vi "Save Image.vi"(8 "error in (no error)":errorcluster, 9 "Export Style":enum32{"Raw", "Graph", "Gray"}(radio), 10 "Export Name":string, 11 "Base Graph in":refnum<class "Base Graph.lvclass">) -> (0 "error out":errorcluster, 3 "Base Graph out":refnum<class "Base Graph.lvclass">)   [LabVIEW 2023, in "Base Graph.lvclass"]
uses:
  Base Graph.lvclass
  Base Graph.lvclass/Base Graph.ctl
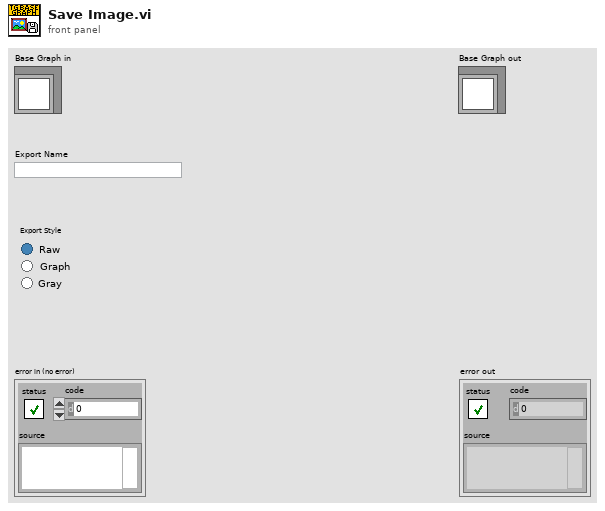
[diagram p1: front panel]
types:
  T1 = typedef "IMAQ Image.ctl" = refnum<image>
  T2 = typedef "imagedata.ctl" = cluster{"image type":i32, "image depth":i32, "image":u8[], "mask":u8[], "colors":u32[], "Rectangle":cluster{"left":i16, "top":i16, "right":i16, "bottom":i16}}
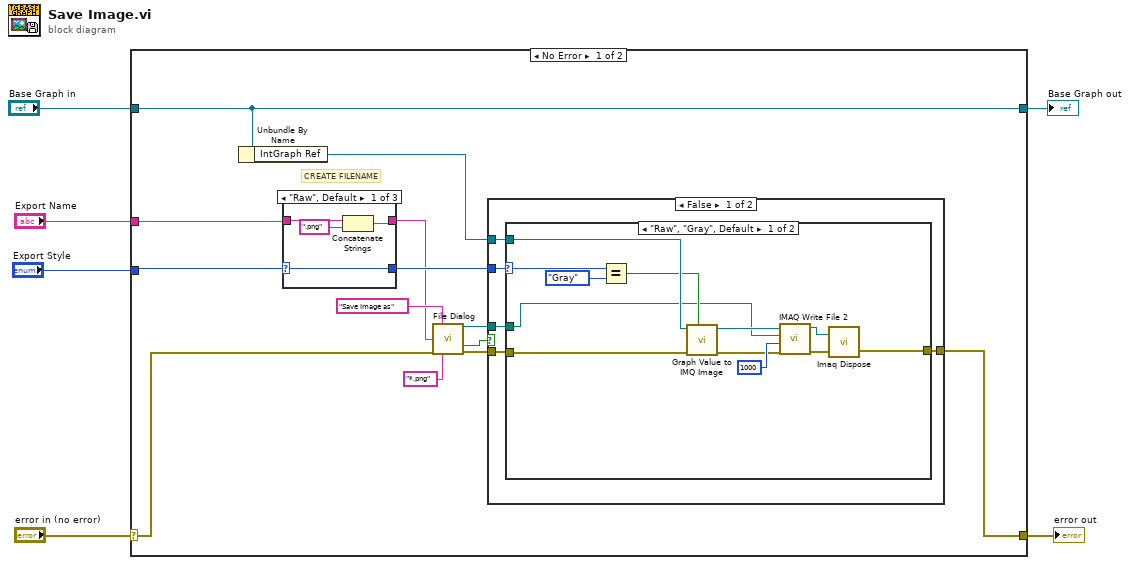
[diagram p0: block diagram]
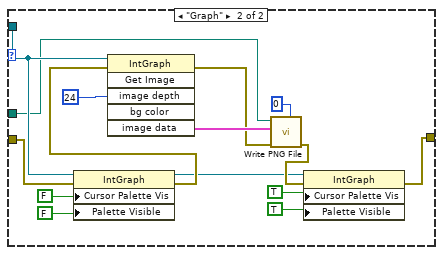
[diagram p2: hidden frame]
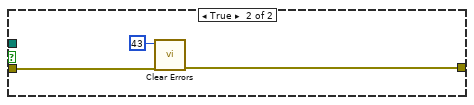
[diagram p3: hidden frame]
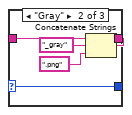
[diagram p4: hidden frame]
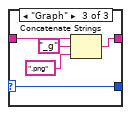
[diagram p5: hidden frame]
diagram:
  n1 = case shown="No Error" "error in (no error)" {
    selector: "error in (no error)" -> [w9 w70]
    tunnel: [w8 w70] -> w5
    tunnel: [w12 w69] -> w3
    tunnel: "Base Graph in" -> [w12 w69]
    tunnel: "Export Name" -> [w10 _]
    tunnel: "Export Style" -> [w7 _]
    frame No Error {
      # "CREATE FILENAME"
      n2 = Unbundle By Name(w12) -> ("IntGraph Ref"=w11:refnum<vi>)
      n3 = case shown="\"Raw\", Default" w7 {
        selector: w7 -> [w58 w61 w68]
        tunnel: [w58 w61 w68] -> w19
        tunnel: w10 -> [w57 w63 w67]
        tunnel: [w55 w62 w64] -> w14
        frame "Raw", Default {
          n4 = Concatenate Strings(w57, ".png" ("string")) -> (w55:string)
        }
        frame "Gray" {
          n5 = Concatenate Strings(w63, "_gray" ("string"), ".png" ("string")) -> (w62:string)
        }
        frame "Graph" {
          n6 = Concatenate Strings(w67, "_g" ("string"), ".png" ("string")) -> (w64:string)
        }
      }
      n7 = call "File Dialog"("prompt"="Save Image as", "default name"=w14, "error in"=w9, "pattern (all files)"="*.png") -> ("selected path"=w13:path, "cancelled"=w15:bool, "error out"=w16:errorcluster)  [unwired: 8 in, 1 out]
      n8 = case shown="False" w15 {
        tunnel: [w24 w53] -> w8
        tunnel: w19 -> [w23 _]
        tunnel: w11 -> [w22 _]
        tunnel: w16 -> [w21 w54]
        tunnel: w13 -> [w20 _]
        frame False {
          n9 = case shown="\"Raw\", \"Gray\", Default" w23 {
            selector: w23 -> [w28 _]
            tunnel: w21 -> [w29 w41]
            tunnel: [w33 w38] -> w24
            tunnel: w22 -> [w30 w40]
            tunnel: w20 -> [w25 w39]
            frame "Raw", "Gray", Default {
              n10 = Equal?(x=w28, y=enum32{"Raw", "Graph", "Gray"}."Gray") -> (x = y?=w26:bool)
              n11 = call "Graph Value to IMQ Image.vi"("Gray?"=w26, "error in"=w29, "Intensity Graph Refnum"=w30) -> ("error out"=w31:errorcluster, "Image Out"=w36:T1)  [unwired: 7 in]
              n12 = call-poly "IMAQ Write File 2"("error in (no error)"=w31, "Image Quality"=u32 1000, "File Path"=w25, "Image"=w36) -> ("error out"=w34:errorcluster, "Image Out (duplicate)"=w35:T1)  [unwired: 6 in]
              n13 = call "Imaq Dispose"("Image"=w35, "error in (no error)"=w34) -> ("error out"=w33:errorcluster)  [unwired: 4 in]
            }
            frame "Graph" {
              n14 = property class="IntGraph"(reference=w40, error in=w41, "Cursor Palette Vis"=FALSE ("Cursor Legend Visible"), "Palette Visible"=FALSE ("Palette:Visible")) -> (reference out=w45:refnum<vi>, error out=w48:errorcluster)
              n15 = invoke class="IntGraph" method="Get Image"(reference=w40, error in=w48, "image depth"=24 ("Image Depth")) -> (error out=w49:errorcluster, "image data"=w50:T2)  [unwired: 3 in, 4 out]
              n16 = call <vilib>:"Write PNG File.vi"("compression (default)"=0, "error in (no error)"=w49, "image data"=w50, "path to PNG file"=w39) -> ("error out"=w46:errorcluster)  [unwired: 6 in, 1 out]
              n17 = property class="IntGraph"(reference=w45, error in=w46, "Cursor Palette Vis"=TRUE ("Cursor Legend Visible"), "Palette Visible"=TRUE ("Palette:Visible")) -> (error out=w38:errorcluster)  [unwired: 1 out]
            }
          }
        }
        frame True {
          n18 = call <vilib>:"Clear Errors.vi"("error in (no error)"=w54, "specific error code to clear (0: all)"=43) -> ("error out"=w53:errorcluster)  [unwired: 4 in, 1 out]
        }
      }
    }
    frame Error {
    }
  }
  "error out" <- w5
  "Base Graph out" <- w3
